vi "Read Mark Values.vi"(8 "error in (no error)":errorcluster, 10 "Channel (0: Channel 1)":i32(ring) items=["Channel 1", "Channel 2", "Channel 3", "Channel 4", "Math", "Bus 1", "Bus 2", "Bus 3", "Bus 4", "Reference 1", "Reference 2", "Reference 3", "Reference 4", "Column", "Digital"], 11 "VISA resource name":refnum<visa-resource-name>) -> (0 "error out":errorcluster, 2 "Marks Array (2D Dbl)":dbl[][](array[numeric]), 3 "VISA resource name out":refnum<visa-resource-name>)   [LabVIEW 2016, in "Tektronix DPO MSO 2000 4000 Series.lvlib"]
doc: "Reads the x and y values off of the marks on time domain channels. Returns an array of these x,y values with one for each mark.\n\n<B>Note:</B>\nValid only in VIs where advanced marks are available. This includes the <B>MDO</B> series and the <B>MSO/DPO 4000B</B> series."
uses:
  Tektronix DPO MSO 2000 4000 Series.lvlib
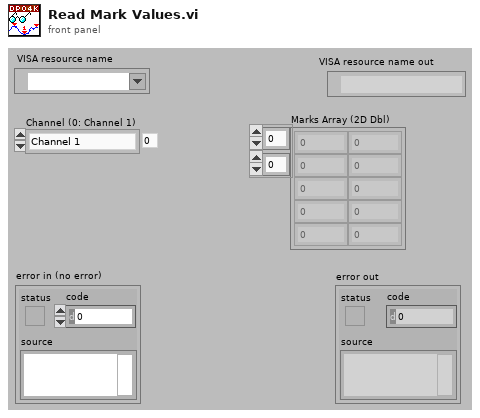
[diagram p1: front panel]
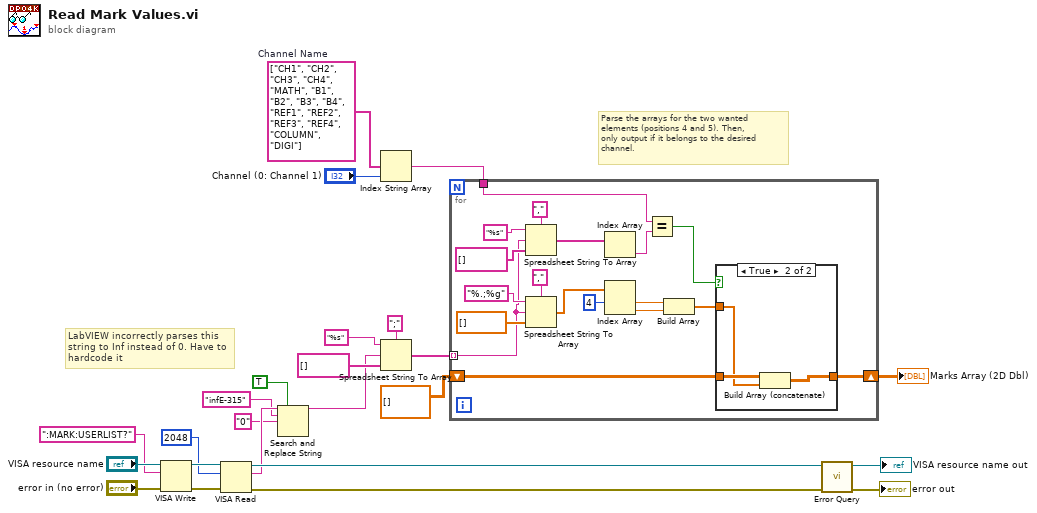
[diagram p0: block diagram]
diagram:
  w10 = string[] ["CH1", "CH2", "CH3", "CH4", "MATH", "B1", "B2", "B3", "B4", "REF1", "REF2", "REF3", "REF4", "COLUMN", "DIGI"]  # Channel Name
  # "LabVIEW incorrectly parses this \nstring to Inf instead of 0. Have to \nhardcode it"
  # "Parse the arrays for the two wanted \nelements (positions 4 and 5). Then,\nonly output if it belongs to the desired \nchannel."
  n1 = VISA Write(VISA resource name="VISA resource name", write buffer=":MARK:USERLIST?", error in (no error)="error in (no error)") -> (VISA resource name out=w20:refnum<visa-resource-name>, error out=w21:errorcluster)  [unwired: 1 out]
  n2 = VISA Read(VISA resource name=w20, byte count=u32 2048, error in (no error)=w21) -> (VISA resource name out=w17:refnum<visa-resource-name>, read buffer=w7:string, error out=w18:errorcluster)  [unwired: 1 out]
  n3 = Search and Replace String(replace all?=TRUE ("replace all? (F)"), input string=w7, search string="infE-315", replace string="0" ("replace string (\"\")")) -> (result string=w4:string)  [unwired: 4 in, 3 out]
  n4 = Index String Array(1:"Channel (0: Channel 1)", 2:w10) -> (0:w8:string)  [unwired: 1 in]
  n5 = Spreadsheet String To Array(delimiter (Tab)=";", format string="%s", spreadsheet string=w4, array type (2D Dbl)=string[] []) -> (array=w11:string[])
  n6 = for {
    tunnel: w11 -> [w33] mode=indexing
    tunnel: w8 -> [w29]
    shift-right: [w25] -> w1
    shift-left: dbl[][] [] ("array type (2D Dbl)") -> [w26]
    n7 = Spreadsheet String To Array(delimiter (Tab)=",", format string="%s" ("spreadsheet string"), spreadsheet string=w33, array type (2D Dbl)=string[] []) -> (array=w32:string[])
    n8 = Spreadsheet String To Array(delimiter (Tab)=",", format string="%.;%g", spreadsheet string=w33, array type (2D Dbl)=dbl[] []) -> (array=w37:dbl[])
    n9 = Index Array(array=w32) -> (element=w31:string)  [unwired: 1 in]
    n10 = Index Array(array=w37, index #1=4 ("index")) -> (element #1=w40:dbl, element #2=w41:dbl)  [unwired: 1 in]
    n11 = Equal?(x=w29, y=w31) -> (x = y?=w28:bool)
    n12 = Build Array(w40, w41) -> (w27:dbl[])
    n13 = case shown="True" w28 {
      tunnel: w27 -> [_ w45]
      tunnel: w26 -> [w43 w46]
      tunnel: [w43 w44] -> w25
      frame False {
      }
      frame True {
        n14 = Build Array (concatenate)(w46, w45) -> (w44:dbl[][])
      }
    }
  }
  "Marks Array (2D Dbl)" <- w1
  n15 = call "Error Query.vi"("error in (no error)"=w18, "VISA resource name"=w17) -> ("error out"=→"error out":errorcluster, "VISA resource name out"=→"VISA resource name out":refnum<visa-resource-name>)  [unwired: 6 in, 2 out]
